vi "erForceSimulatorPackage.vi"(8 "error in (no error)":errorcluster, 10 "robots":T1[](array[typedef]), 11 "Communication in":refnum<class "Communication.lvclass">) -> (0 "error out":errorcluster, 2 "robotControl":u8[](array[numeric]), 3 "Communication out":refnum<class "Communication.lvclass">)   [LabVIEW 2023, in "Communication.lvclass"]
uses:
  Communication.lvclass
  Convert AI Robot to Robot Command Folder/grSim/grSim Robot Command.ctl
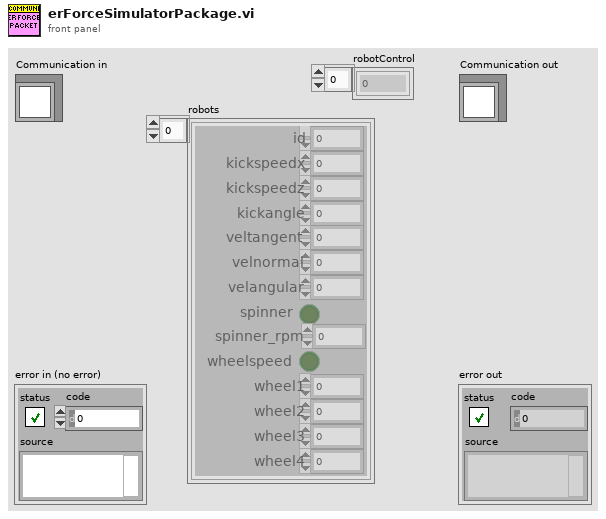
[diagram p1: front panel]
types:
  T1 = typedef "grSim Robot Command.ctl" = cluster{"id":u32, "kickspeedx":sgl, "kickspeedz":sgl, "veltangent":sgl, "velnormal":sgl, "velangular":sgl, "spinner":bool, "wheelspeed":bool, "wheel1":sgl, "wheel2":sgl, "wheel3":sgl, "wheel4":sgl, "kickangle":sgl, "spinner_rpm":sgl}
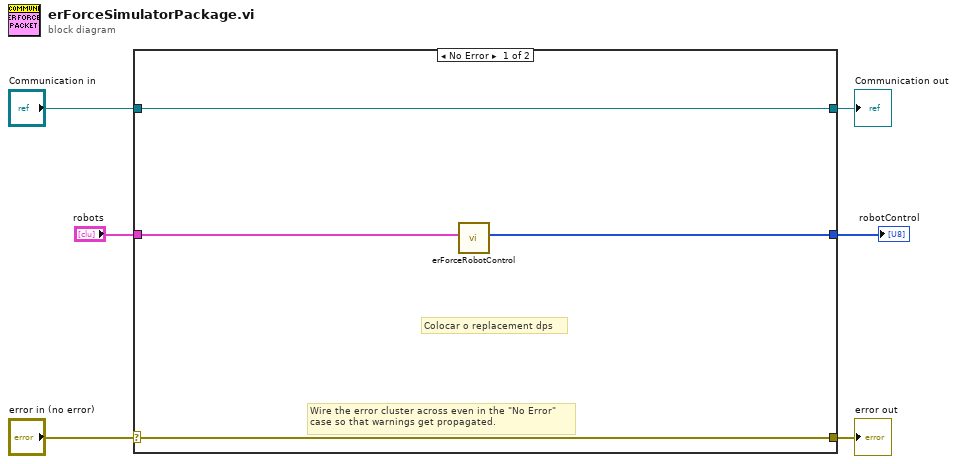
[diagram p0: block diagram]
diagram:
  n1 = case shown="No Error" "error in (no error)" {
    selector: "error in (no error)" -> [w9 w12]
    tunnel: [w9 w12] -> w5
    tunnel: [w10 w11] -> w3
    tunnel: "Communication in" -> [w10 w11]
    tunnel: [w8 _] -> w2
    tunnel: "robots" -> [w7 _]
    frame No Error {
      # "Colocar o replacement dps"
      # "Wire the error cluster across even in the \"No Error\"\ncase so that warnings get propagated."
      n2 = call "erForceRobotControl.vi"("robots"=w7) -> ("robotControl"=w8:u8[])  [unwired: 8 in, 2 out]
    }
    frame Error {
    }
  }
  "error out" <- w5
  "Communication out" <- w3
  "robotControl" <- w2
